vi "Write Data_HoldingRegistors.vi"(6 "Index":i32, 8 "error in (no error)":errorcluster, 9 "register values":dbl[](array[numeric]), 11 "Device in":refnum<class "MB_TCP_Device.lvclass">) -> (0 "error out":errorcluster, 3 "Device out":refnum<class "MB_TCP_Device.lvclass">)   [LabVIEW 2023, in "MB_TCP_Device.lvclass"]
uses:
  MB_TCP_Device.lvclass
  MB_TCP_Device.lvclass/MB_TCP_Device.ctl
  <vilib>/NI Modbus.llb/MB Ethernet Master Query Write Multiple Registers (poly).vi
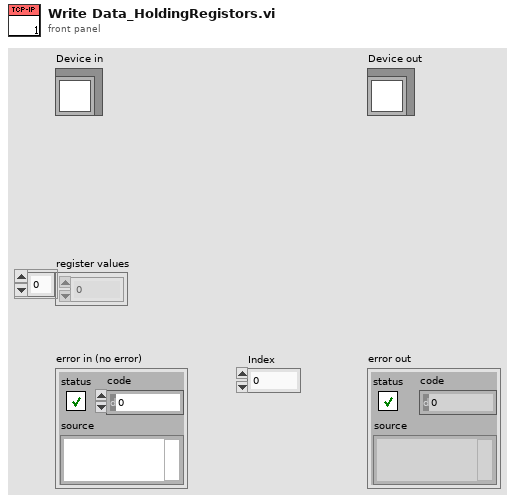
[diagram p1: front panel]
types:
  T1 = typedef "DAQ Device_IO ChannelsData.ctl" = cluster{"#DigitalInputs":u16, "StartAddress_DI":u16, "#DigitalOutputs":u16, "StartAddress_DO":u16, "#AnalogInputs":u16, "StartAddress_AI":u16, "#AnalogOutputs":u16, "StartAddress_AO":u16, "Coil_ReadData":bool[], "Coil_WriteData":bool[], "AI_Data":u16[], "AO_Data":u16[]}
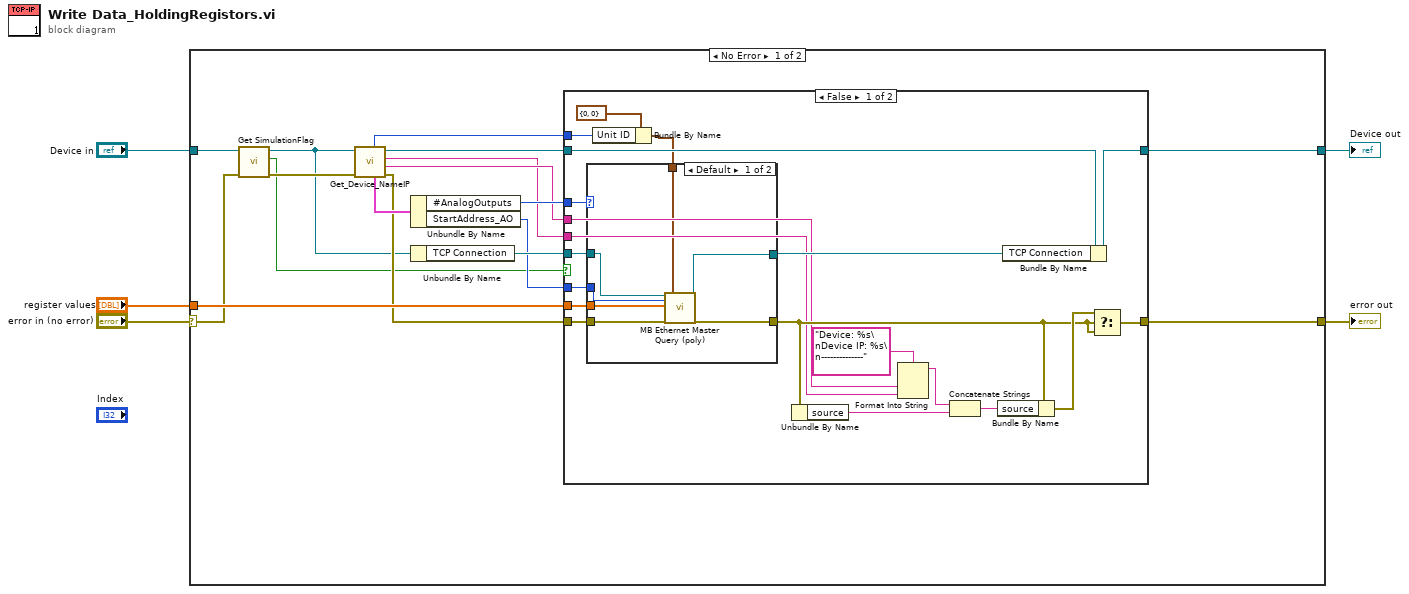
[diagram p0: block diagram]
diagram:
  n1 = case shown="No Error" "error in (no error)" {
    selector: "error in (no error)" -> [w9 w55]
    tunnel: [w21 w55] -> w4
    tunnel: [w19 w54] -> w2
    tunnel: "Device in" -> [w12 w54]
    tunnel: "register values" -> [w22 _]
    frame No Error {
      n2 = call-dynamic "Get SimulationFlag.vi"("error in (no error)"=w9, "Device in"=w12) -> ("error out"=w10:errorcluster, "Simulation?"=w7:bool, "Device out"=w6:refnum<class "MB_TCP_Device.lvclass">)  [unwired: 7 in]
      n3 = call-dynamic "Get_Device_NameIP.vi"("error in (no error)"=w10, "Device in"=w6) -> ("error out"=w8:errorcluster, "Device Name"=w14:string, "Device Address"=w13:string, "Device out"=w17:refnum<class "MB_TCP_Device.lvclass">, "IO Channels"=w18:T1, "Unit ID"=w11:u8)  [unwired: 4 in]
      n4 = Unbundle By Name(w18) -> ("#AnalogOutputs"=w16:u16, "StartAddress_AO"=w15:u16)
      n5 = Unbundle By Name(w6) -> ("TCP Connection"=w20:refnum<k5>)
      n6 = case shown="False" w7 {
        tunnel: [w42 w53] -> w19
        tunnel: w8 -> [w40 w52]
        tunnel: w15 -> [w39 _]
        tunnel: w22 -> [w27 _]
        tunnel: [w36 w52] -> w21
        tunnel: w20 -> [w35 _]
        tunnel: w13 -> [w33 _]
        tunnel: w17 -> [w31 w53]
        tunnel: w14 -> [w30 _]
        tunnel: w16 -> [w26 _]
        tunnel: w11 -> [w23 _]
        frame False {
          n7 = Bundle By Name(cluster=cluster{"Transaction ID":u16, "Unit ID":u8} {"Transaction ID"=0, "Unit ID"=0} ("MBAP Header"), "Unit ID"=w23) -> (w24:cluster{"Transaction ID":u16, "Unit ID":u8})
          n8 = case shown="Default" w26 {
            tunnel: [w49 w51] -> w41
            tunnel: w40 -> [w48 w50]
            tunnel: w39 -> [w47 _]
            tunnel: [w46 w50] -> w37
            tunnel: w35 -> [w45 w51]
            tunnel: w27 -> [w44 _]
            tunnel: w24 -> [w43 _]
            frame Default {
              n9 = call-poly <vilib>:"MB Ethernet Master Query (poly).vi"("TCP Connection Refnum in"=w45, "Starting Address"=w47, "Registers"=w44, "error in"=w48, "MBAP Header"=w43) -> ("TCP Connection Refnum (dup)"=w49:refnum<k5>, "error out"=w46:errorcluster)  [unwired: 12 in, 1 out]
            }
            frame 0 {
            }
          }
          n10 = Unbundle By Name(w37) -> ("source"=w34:string)
          n11 = Format Into String(format string="Device: %s\nDevice IP: %s\n--------------", w30, w33) -> (resulting string=w29:string)  [unwired: 2 in, 1 out]
          n12 = Concatenate Strings(w29, w34) -> (w28:string)
          n13 = Bundle By Name(cluster=w37, "source"=w28) -> (w38:errorcluster)
          n14 = Bundle By Name(cluster=w31, "TCP Connection"=w41) -> (w42:refnum<class "MB_TCP_Device.lvclass">)
          n15 = Select(t=w38, s=w37, f=w37) -> (s? t:f=w36:errorcluster)
        }
        frame True {
        }
      }
    }
    frame Error {
    }
  }
  "error out" <- w4
  "Device out" <- w2
